vi "Validate PCL Decimation Value.vi"(7 "PCL Decimation":u32, 8 "Error In":errorcluster, 11 "Instrument Addon Refnum In":T1 format="%.0x") -> (0 "Error Out":errorcluster, 3 "Instrument Addon Refnum Out":T1 format="%.0x")   [LabVIEW 2019, in "Instrument Addon Scripting API.lvlib"]
doc: "Verifies if the PCL Decimation value is greater or equal than 1\n\nInput\nPCL Decimation: the PCL Decimation value specified by the user.\nInstrument Addon Refnum In: the reference number of to the Instrument Addun Custom Device of which PCL Rate is about to be set.\n\nOutput: \nInstrument Addon Refnum Out: the reference number to the Instrument Addon Custom Device provided as input"
uses:
  Instrument Addon Scripting API.lvlib
  <vilib>/NI VeriStand/Custom Device API/Custom Device Item Ref.ctl
  <vilib>/NI VeriStand/Custom Device API/Custom Device API.lvlib
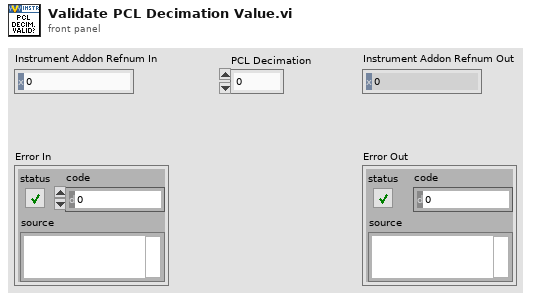
[diagram p1: front panel]
types:
  T1 = typedef "Custom Device API.lvlib/Custom Device Item Ref.ctl" = u64
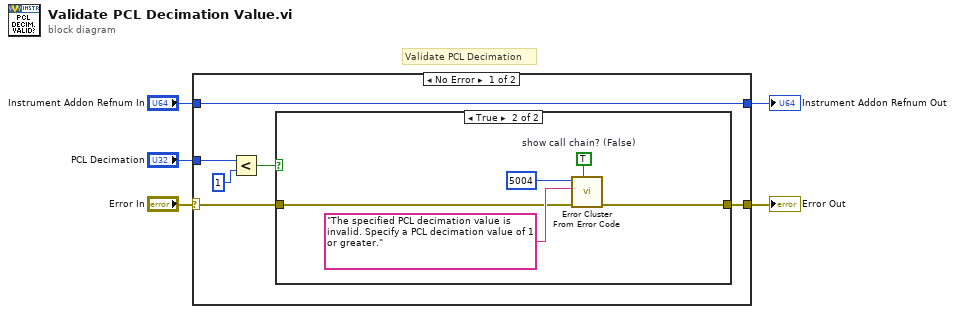
[diagram p0: block diagram]
diagram:
  # "Validate PCL Decimation"
  n1 = case shown="No Error" "Error In" {
    selector: "Error In" -> [w8 w19]
    tunnel: "PCL Decimation" -> [w10 _]
    tunnel: [w7 w19] -> w3
    tunnel: "Instrument Addon Refnum In" -> [w6 w18]
    tunnel: [w6 w18] -> w1
    frame No Error {
      n2 = Less?(x=w10, y=u32 1) -> (x < y?=w9:bool)
      n3 = case shown="True" w9 {
        tunnel: w8 -> [w12 w14]
        tunnel: [w12 w17] -> w7
        frame False {
        }
        frame True {
          w13 = TRUE  # show call chain? (False)
          n4 = call <vilib>:"Error Cluster From Error Code.vi"("show call chain? (False)"=w13, "error in (no error)"=w14, "error message (\"\")"="The specified PCL decimation value is invalid. Specify a PCL decimation value of 1 or greater." ("error message (\"\")"), "error code (0)"=5004) -> ("error out"=w17:errorcluster)  [unwired: 5 in]
        }
      }
    }
    frame Error {
    }
  }
  "Error Out" <- w3
  "Instrument Addon Refnum Out" <- w1
